vi "Write N.vi"(8 "error in (no error)":errorcluster, 10 "N":i32, 11 "MB_TCP in":refnum<class "MB_TCP.lvclass">) -> (0 "error out":errorcluster, 3 "MB_TCP out":refnum<class "MB_TCP.lvclass">)   [LabVIEW 2019, in "MB_TCP.lvclass"]
uses:
  MB_TCP.lvclass
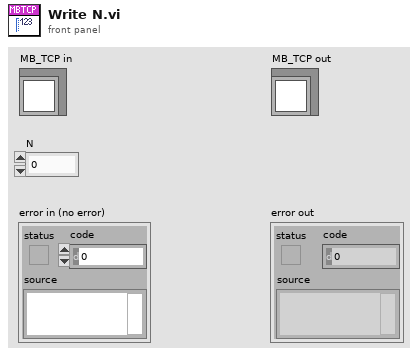
[diagram p1: front panel]
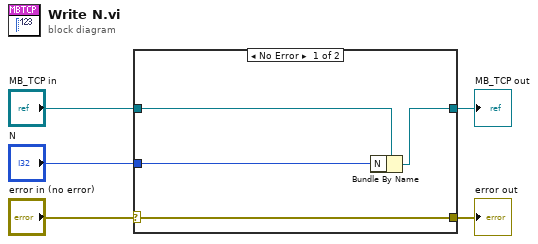
[diagram p0: block diagram]
diagram:
  n1 = case shown="No Error" "error in (no error)" {
    selector: "error in (no error)" -> [w9 w11]
    tunnel: [w9 w11] -> w4
    tunnel: [w7 w10] -> w2
    tunnel: "MB_TCP in" -> [w8 w10]
    tunnel: "N" -> [w6 _]
    frame No Error {
      n2 = Bundle By Name(cluster=w8, "N"=w6) -> (w7:refnum<class "MB_TCP.lvclass">)
    }
    frame Error {
    }
  }
  "error out" <- w4
  "MB_TCP out" <- w2
